vi "Create Name Msg Output Refs.vi"(6 "Name Msg":string, 8 "error in":errorcluster, 9 "Name Library File Path":path, 10 "Active Project":refnum<vi>) -> (0 "error out":errorcluster, 2 "Name Msg Output Refs":T1)   [LabVIEW 2025, in "_Rescript.lvlib" / "_Rescript.lvclass"]
uses:
  _Rescript.lvclass
  Name Msg Output Refs.ctl
  <vilib>/Utility/traverseref.llb/TRef TravTarget.ctl
  _Rescript.lvclass/_Rescript.ctl
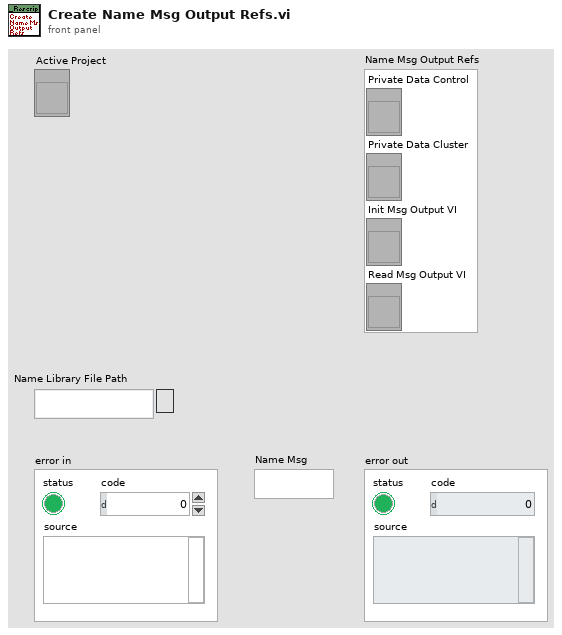
[diagram p1: front panel]
types:
  T1 = typedef "_Rescript.lvlib/_Rescript.lvclass/Name Msg Output Refs.ctl" = cluster{"Private Data Control":refnum<vi>, "Private Data Cluster":refnum<vi>, "Init Msg Output VI":refnum<vi>, "Read Msg Output VI":refnum<vi>}
  T2 = typedef "TRef TravTarget.ctl" = enum16{"FP", "BD", "Other"}
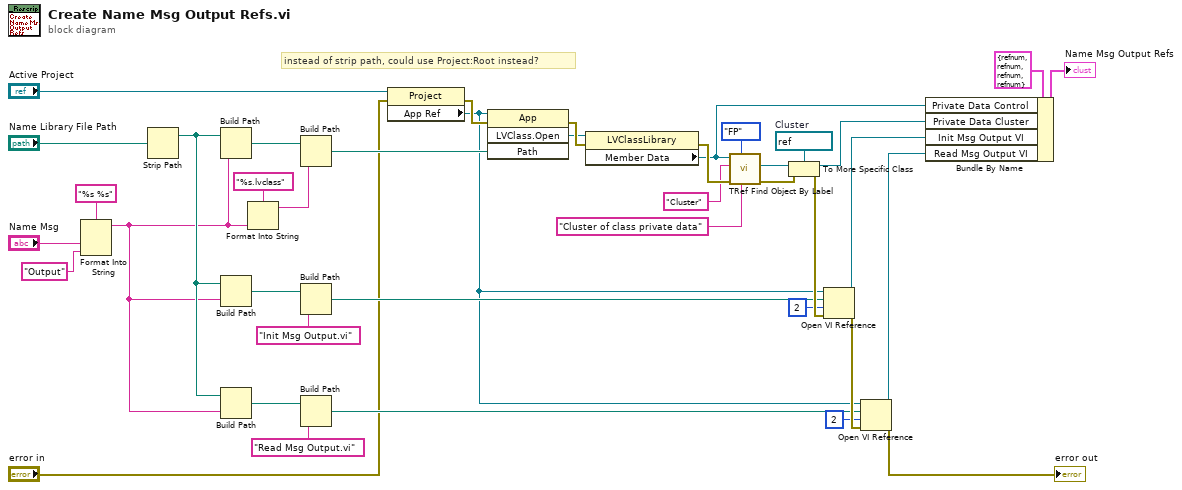
[diagram p0: block diagram]
diagram:
  w34 = refnum<vi> refnum  # Cluster
  # "instead of strip path, could use Project:Root instead?"
  n1 = Format Into String(format string="%s %s", "Name Msg", "Output" ("input 6")) -> (resulting string=w3:string)  [unwired: 2 in, 1 out]
  n2 = Strip Path(path="Name Library File Path") -> (stripped path=w14:path)  [unwired: 1 out]
  n3 = Build Path(base path=w14, name or relative path=w3) -> (appended path=w28:path)
  n4 = Build Path(base path=w14, name or relative path=w3) -> (appended path=w24:path)
  n5 = Build Path(base path=w14, name or relative path=w3) -> (appended path=w23:path)
  n6 = Format Into String(format string="%s.lvclass", w3) -> (resulting string=w26:string)  [unwired: 2 in, 1 out]
  n7 = Build Path(base path=w28, name or relative path=w26) -> (appended path=w27:path)
  n8 = Build Path(base path=w24, name or relative path="Init Msg Output.vi" ("format string")) -> (appended path=w20:path)
  n9 = Build Path(base path=w23, name or relative path="Read Msg Output.vi" ("format string")) -> (appended path=w19:path)
  n10 = property class="Project"(reference="Active Project", error in="error in") -> (error out=w38:errorcluster, "App Ref"=w13:refnum<vi>)  [unwired: 1 out]
  n11 = invoke class="App" method="LVClass.Open"(reference=w13, error in=w38, "Path"=w27) -> (error out=w36:errorcluster, "LVClass.Open"=w29:refnum<vi>)  [unwired: 1 in, 2 out]
  n12 = property class="LVClassLibrary"(reference=w29, error in=w36) -> (error out=w40:errorcluster, "Member Data"=w12:refnum<vi>)  [unwired: 1 out]
  n13 = call <vilib>:"TRef Find Object By Label.vi"("Label"="Cluster of class private data" ("Class Name"), "Traverse Target"=TRef_TravTarget."FP", "error in (no error)"=w40, "Class Name"="Cluster", "VI Ref"=w12) -> ("error out"=w35:errorcluster, "Found Obj Ref"=w33:refnum<vi>)  [unwired: 3 in, 2 out]
  n14 = To More Specific Class(target class=w34, reference=w33, error in=w35) -> (specific class reference=w11:refnum<vi>, error out=w37:errorcluster)
  n15 = Open VI Reference(application reference (local)=w13, vi path=w20, options=2, error in (no error)=w37) -> (vi reference=w10:refnum<vi>, error out=w39:errorcluster)  [unwired: 2 in]
  n16 = Open VI Reference(application reference (local)=w13, vi path=w19, options=2, error in (no error)=w39) -> (vi reference=w9:refnum<vi>, error out=→"error out":errorcluster)  [unwired: 2 in]
  n17 = Bundle By Name(cluster=T1 {"Private Data Control"=refnum, "Private Data Cluster"=refnum, "Init Msg Output VI"=refnum, "Read Msg Output VI"=refnum} ("Name Msg Output Refs"), "Private Data Control"=w12, "Private Data Cluster"=w11, "Init Msg Output VI"=w10, "Read Msg Output VI"=w9) -> (→"Name Msg Output Refs":T1)
